vi "VEHICLE MODEL CAN1.vi"() -> ()   [LabVIEW 2015]
uses:
  <vilib>/Platform/TimedLoop/XDataNode/timing_clust.ctl
  <vilib>/Platform/TimedLoop/XDataNode/nitl_modes.ctl
  <vilib>/Platform/TimedLoop/XDataNode/wakeup.ctl
  <vilib>/FPGAPlugInAG/cRIO-9063/niLvFpga_Open_cRIO-9063.vi
  <vilib>/rvi/interface/common/dynamic/niFpgaDynamicAddResources.vi
  <vilib>/Utility/error.llb/Error Cluster From Error Code.vi
  <vilib>/rvi/errors/niLvFpgaAdjustHostInterfaceError.vi
  <vilib>/FPGAPlugInAG/Dynamic/niLvFpga_Close_Dynamic.vi
  <vilib>/rvi/interface/nirviOpenFPGA/nirviOpenFPGA.xnode
  FPGA Bitfiles/VCU-VEHICLEMODEL_FPGATarget_CANBasic(FPGA)_WVt1gIpoBPw.lvbitx
  Basic (FPGA) CAN Engine .vi
  <vilib>/Platform/TimedLoop/XDataNode/XDataNode.xnode
  <vilib>/rvi/interface/nirviReadWriteControl/nirviReadWriteControl.xnode
  <vilib>/rvi/interface/nirviCloseFPGA/nirviCloseFPGA.xnode
  <vilib>/Platform/TimedLoop/XDataNode/XDNodeRunTimeDep.lvlib
  <vilib>/rvi/interface/Simulation/niFpgaSimulationCallBeginRW.vi
  NiFpgaLv.dll
panel:
  out "Old Timestamp":u64
  out "Current Timestamp":u64
  out "?":cluster{dbl, dbl}[](graph)
  out "F":dbl
  out "Theta":dbl
  in  "?":bool
  in  "RUNNING":bool
  out "Vy":dbl
  out "Vx":dbl
  out "Py":dbl
  out "Px":dbl
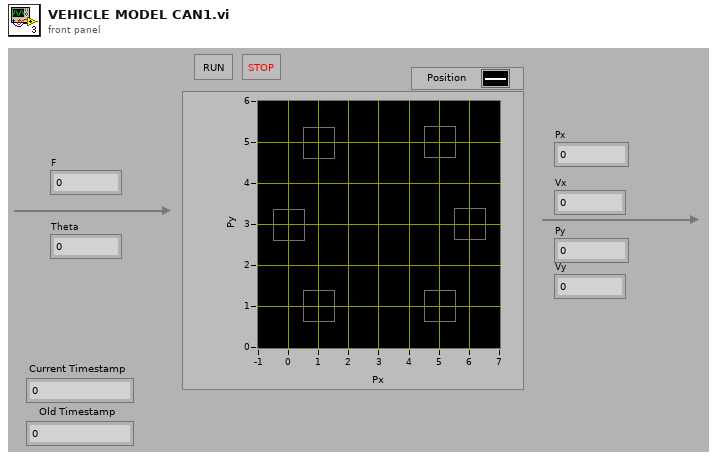
[diagram p1: front panel]
types:
  T1 = typedef "XDNodeRunTimeDep.lvlib/timing_clust.ctl" = cluster{"Expected End [f-1]":u64, "Actual End [f-1]":u64, "Finished Late? [f-1]":bool, "Expected End [i-1]":u64, "Actual End [i-1]":u64, "Finished Late? [i-1]":bool, "Expected Start [i]":u64, "Actual Start [i]":u64, "Expected Start [f]":u64, "Actual Start [f]":u64, "Source Name":string, "Structure Name":string, "Period":i64, "Deadline":i64, "Offset":i64, "Start":i64, "Priority":i32, "Timeout":i32, "Mode":T2, "Wakeup Reason":T3, "Error":errorcluster, "Source Type":string, "Secondary Source Type":string, "Global End Time":u64, "Global Start Time":u64, "Frame Duration":u64, "Iteration Duration":u64, "Assigned CPU":i32, "I/O Scan Engine Mode":u32}
  T2 = typedef "XDNodeRunTimeDep.lvlib/nitl_modes.ctl" = enum32{"No Change", "Process missed periods, maintain original phase", "Discard missed periods, maintain original phase", "Process missed periods, ignore original phase", "Discard missed periods, ignore original phase"}
  T3 = typedef "XDNodeRunTimeDep.lvlib/wakeup.ctl" = enum32{"Normal", "Aborted", "Asynchronous wakeup", "Timing source error", "Timed loop error", "Timeout"}
  T4 = cluster{"timestamp high":u32, "timestamp low":u32, "identifier":u32, "type":enum8{"Data Frame", "Remote Frame", "(reserved)", "(reserved) ", "(reserved)  ", "(reserved)   ", "Bus Error", "Transceiver Fault"}, "info A":u8, "info B":u8, "data length":u8, "data":u8[]}
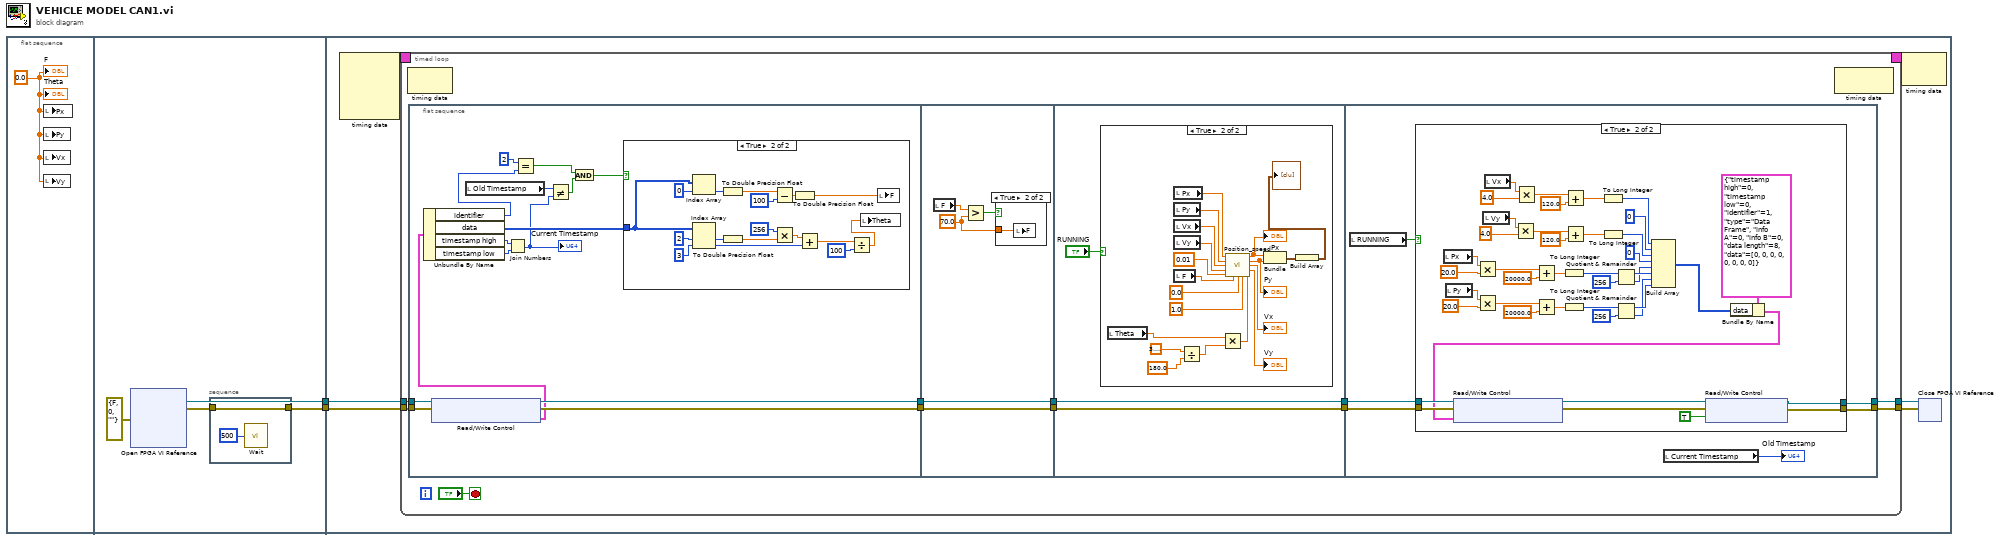
[diagram p0: block diagram]
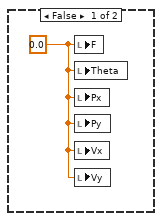
[diagram p4: hidden frame]
diagram:
  n1 = flat-sequence {
    tunnel: [w6] -> w2
    tunnel: [w4] -> w1
    tunnel: w2 -> [w13]
    tunnel: w1 -> [w12]
    frame #0 {
      w3 = 0.0 ("F")
      n2 = local write "Px"(w3) -> ()
      n3 = local write "Py"(w3) -> ()
      n4 = local write "Vx"(w3) -> ()
      n5 = local write "Vy"(w3) -> ()
      "Theta" <- w3
      "F" <- w3
    }
    frame #1 {
      n6 = xnode "Open FPGA VI Reference"("error in"=errorcluster {"status"=FALSE, "code"=0, "source"=""}) -> ("FPGA VI Reference Out"=w6:refnum<k20>, "error out"=w5:errorcluster)  [unwired: 1 in]
      n7 = stacked-sequence {
        tunnel: w5 -> [w9]
        tunnel: [w9] -> w4
        frame #0 {
          n8 = call "Wait"("Count(mSec)"=u32 500) -> ()  [unwired: 1 out]
        }
      }
    }
    frame #2 {
      n9 = node-c288() -> (w15:T1)  [unwired: 4 in]
      n10 = timed-loop {
        timing: w15 -> [_]
        timing-out: [_] -> w14
        tunnel: [w24] -> w11
        tunnel: w13 -> [w23]
        tunnel: w12 -> [w22]
        tunnel: [w20] -> w10
        stop <- "?" stop-if-true
        n11 = node-c288() -> ()  [unwired: 1 in, 1 out]
        n12 = flat-sequence {
          tunnel: [w43] -> w19
          tunnel: w23 -> [w42]
          tunnel: w22 -> [w41]
          tunnel: [w40] -> w17
          tunnel: w19 -> [w65]
          tunnel: [w65] -> w18
          tunnel: w17 -> [w64]
          tunnel: [w64] -> w16
          tunnel: [w69] -> w25
          tunnel: w18 -> [w69]
          tunnel: [w68] -> w21
          tunnel: w16 -> [w68]
          tunnel: w25 -> [w95]
          tunnel: [w93] -> w24
          tunnel: w21 -> [w94]
          tunnel: [w92] -> w20
          frame #0 {
            n13 = xnode "Read/Write Control"("FPGA VI Reference In"=w42, "error in"=w41) -> ("FPGA VI Reference Out"=w43:refnum<k20>, "error out"=w40:errorcluster, "CAN1 - Received Frame"=w37:T4)
            n14 = Unbundle By Name(w37) -> ("identifier"=w32:u32, "data"=w39:u8[], "timestamp high"=w36:u32, "timestamp low"=w35:u32)
            n15 = local read "Old Timestamp"() -> (w34:u64)
            n16 = Join Numbers(hi=w36, lo=w35) -> ((hi.lo)=w33:u64)
            "Current Timestamp" <- w33
            n17 = Equal?(x=u32 2 ("y"), y=w32) -> (x = y?=w30:bool)
            n18 = Not Equal?(x=w34, y=w33) -> (x != y?=w31:bool)
            n19 = And(x=w30, y=w31) -> (x .and. y?=w29:bool)
            n20 = case shown="True" w29 {
              tunnel: w39 -> [_ w57]
              frame False {
              }
              frame True {
                n21 = Index Array(array=w57, index=0 ("索引")) -> (element=w47:u8)
                n22 = Index Array(array=w57, index #1=2 ("索引"), index #2=3 ("索引")) -> (element #1=w48:u8, element #2=w53:u8)
                n23 = To Double Precision Float(number=w47) -> (double precision float=w46:dbl)
                n24 = To Double Precision Float(number=w48) -> (double precision float=w49:dbl)
                n25 = Subtract(x=w46, y=u32 100) -> (x-y=w50:dbl)
                n26 = Multiply(x=u32 256 ("y"), y=w49) -> (x*y=w54:dbl)
                n27 = To Double Precision Float(number=w50) -> (double precision float=w44:dbl)
                n28 = Add(x=w54, y=w53) -> (x+y=w51:dbl)
                n29 = Divide(x=w51, y=u32 100) -> (x/y=w45:dbl)
                n30 = local write "Theta"(w45) -> ()
                n31 = local write "F"(w44) -> ()
              }
            }
          }
          frame #1 {
            w61 = 70.0 ("y")
            n32 = local read "F"() -> (w63:dbl)
            n33 = Greater?(x=w63, y=w61) -> (0:w62:bool)
            n34 = case shown="True" w62 {
              tunnel: w61 -> [_ w66]
              frame False {
              }
              frame True {
                n35 = local write "F"(w66) -> ()
              }
            }
          }
          frame #2 {
            n36 = case shown="True" "RUNNING" {
              frame False {
                w70 = 0.0 ("Theta")
                n37 = local write "F"(w70) -> ()
                n38 = local write "Theta"(w70) -> ()
                n39 = local write "Px"(w70) -> ()
                n40 = local write "Py"(w70) -> ()
                n41 = local write "Vx"(w70) -> ()
                n42 = local write "Vy"(w70) -> ()
              }
              frame True {
                n43 = local read "Theta"() -> (w72:dbl)
                n44 = local read "Px"() -> (w85:dbl)
                n45 = local read "Py"() -> (w84:dbl)
                n46 = local read "Vx"() -> (w83:dbl)
                n47 = local read "Vy"() -> (w82:dbl)
                n48 = local read "F"() -> (w80:dbl)
                n49 = Divide(x=3.141592653589793, y=180.0) -> (x/y=w71:dbl)
                n50 = Multiply(x=w72, y=w71) -> (x*y=w81:dbl)
                n51 = call "Position_speed.vi"("Px"=w85, "Py"=w84, "Vx"=w83, "Vy"=w82, "Delta_T"=0.01 ("F"), "F"=w80, "f"=0.0, "m"=1.0, "Theta"=w81) -> ("Px"=w78:dbl, "Py"=w77:dbl, "Vx"=→"Vx":dbl, "Vy"=→"Vy":dbl)  [unwired: 3 in]
                "Px" <- w78
                "Py" <- w77
                n52 = Bundle("Px"=w78, "Py"=w77) -> (w76:cluster{"Px":dbl, "Py":dbl})  [unwired: 1 in]
                n53 = Build Array(w76) -> (→"?":cluster{"Px":dbl, "Py":dbl}[])
              }
            }
          }
          frame #3 {
            n54 = local read "RUNNING"() -> (w91:bool)
            n55 = case shown="True" w91 {
              tunnel: w95 -> [w97 w139]
              tunnel: w94 -> [w96 w138]
              tunnel: [w97 w134] -> w93
              tunnel: [w96 w133] -> w92
              frame False {
              }
              frame True {
                n56 = local read "Px"() -> (w110:dbl)
                n57 = local read "Py"() -> (w105:dbl)
                n58 = Multiply(x=w110, y=20.0) -> (x*y=w119:dbl)
                n59 = Multiply(x=w105, y=20.0) -> (x*y=w113:dbl)
                n60 = local read "Vy"() -> (w123:dbl)
                n61 = local read "Vx"() -> (w131:dbl)
                n62 = Multiply(x=w123, y=4.0) -> (x*y=w126:dbl)
                n63 = Multiply(x=w131, y=4.0) -> (x*y=w130:dbl)
                n64 = Add(x=w119, y=20000.0) -> (x+y=w117:dbl)
                n65 = Add(x=w113, y=20000.0) -> (x+y=w111:dbl)
                n66 = To Long Integer(number=w117) -> (32bit integer=w122:i32)
                n67 = To Long Integer(number=w111) -> (32bit integer=w116:i32)
                n68 = Add(x=w130, y=120.0) -> (x+y=w128:dbl)
                n69 = Add(x=w126, y=120.0) -> (x+y=w124:dbl)
                n70 = To Long Integer(number=w128) -> (32bit integer=w104:i32)
                n71 = To Long Integer(number=w124) -> (32bit integer=w101:i32)
                n72 = Quotient & Remainder(x=w122, y=256) -> (x-y*floor(x/y)=w109:i32, floor(x/y)=w108:i32)
                n73 = Quotient & Remainder(x=w116, y=256) -> (x-y*floor(x/y)=w107:i32, floor(x/y)=w106:i32)
                n74 = Build Array(w104, 0 ("元素"), w101, 0 ("元素"), w108, w109, w106, w107) -> (w99:i32[])
                n75 = Bundle By Name(cluster=T4 {"timestamp high"=0, "timestamp low"=0, "identifier"=1, "type"=enum."Data Frame", "info A"=0, "info B"=0, "data length"=8, "data"=[0, 0, 0, 0, 0, 0, 0, 0]} ("CAN1 - Transmit Frame"), "data"=w99) -> (w98:T4)
                n76 = xnode "Read/Write Control"("FPGA VI Reference In"=w139, "error in"=w138, "CAN1 - Transmit Frame"=w98) -> ("FPGA VI Reference Out"=w137:refnum<k20>, "error out"=w136:errorcluster)
                n77 = xnode "Read/Write Control"("FPGA VI Reference In"=w137, "error in"=w136, "CAN1 - Transmit"=TRUE) -> ("FPGA VI Reference Out"=w134:refnum<k20>, "error out"=w133:errorcluster)
              }
            }
            n78 = local read "Current Timestamp"() -> (→"Old Timestamp":u64)
          }
        }
        n79 = node-c288() -> ()  [unwired: 1 in, 1 out]
      }
      n80 = node-c288(w14) -> ()  [unwired: 1 out]
      n81 = xnode "Close FPGA VI Reference"("FPGA VI Reference In"=w11, "error in"=w10) -> ()  [unwired: 1 out]
    }
  }
